vi "Unregister Event(All Registers In Customize Event).vi"(8 "error in (no error)":errorcluster, 11 "Event Name":string) -> (0 "error out":errorcluster)   [LabVIEW 2019, in "GaitDAQ UI Event.lvlib"]
uses:
  GaitDAQ UI Event.lvlib
  <userlib>/JUL/Event Message Module/Event Message Library/Event Action.ctl
panel:
  # "Input"
  # "Output"
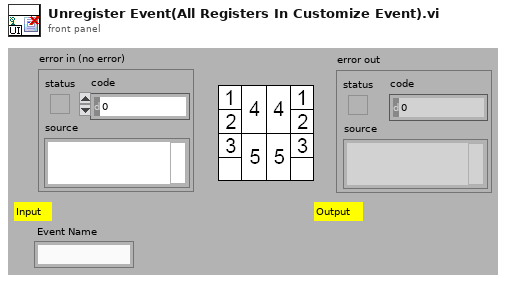
[diagram p1: front panel]
types:
  T1 = typedef "Event Action.ctl" = enum16{"Default", "Generate Event", "Register", "Unregister(Customize Event and Register)", "Unregister(All Events In Customize Register)", "Unregister(All Registers In Customize Event)", "Get Register Table"}
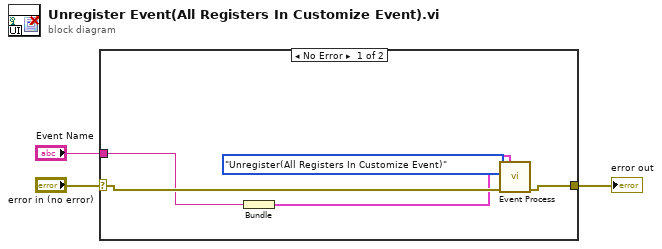
[diagram p0: block diagram]
diagram:
  n1 = case shown="No Error" "error in (no error)" {
    selector: "error in (no error)" -> [w7 w9]
    tunnel: [w6 w9] -> w1
    tunnel: "Event Name" -> [w5 _]
    frame No Error {
      n2 = Bundle("Event Name"=w5) -> (w4:cluster{"Event Name":string})  [unwired: 1 in]
      n3 = call "Event Process.vi"("Event Action"=Event_Action."Unregister(All Registers In Customize Event)", "Unregister Event Data(All Events In Customize Register)"=w4, "error in (no error)"=w7) -> ("error out"=w6:errorcluster)  [unwired: 11 in, 1 out]
    }
    frame Error {
    }
  }
  "error out" <- w1
